vi "AVI Video Conditional Close.vi"(8 "error in (no error)":errorcluster, 11 "Logging queue element in":T1={"Imaging Protocol"=enum."Live Imaging", "Number of Trials"=0, "Frame Size"=512, "# Averaged frames"=0, "Dwell time (us)"=0.0, "Index of Z-plane"=0, "Timelapse?"=FALSE, "Logging process is active"=FALSE, "Speed logging enabled"=FALSE, "tdms file ref"=refnum, "path"=path "", "Trial Number"=0, "Expected # points acquired"=FALSE, "Manually stopped"=FALSE, "Last trial"=FALSE, "Ch0 data"=[], "Ch1 data"=[], "Ref Data"=[], "Ref Frame Time"=[], "Image Time"=[], "Continuous Time"=[], "Ref X Length"=0, "Ref Y Length"=0, "# Ref Averaged frames"=0, "Ref Dwell time (us)"=0.0, "Points acquired"={"Ch0 last trial"=0, "Ch1 last trial"=0, "All trials"=0}, "HW Timings File"=refnum} {"Ref Dwell time (us)" format="%#.6g"; "Frame Size" items=["100X100"=100, "128X128"=128, "200X200"=200, "256X256"=256, "512X512"=512, "1024x1024"=1024, "2048x2048"=2048]; "Dwell time (us)" format="%#.6g"}) -> (0 "error out":errorcluster)   [LabVIEW 2020]
uses:
  Typedefs/Logging queue element.ctl
  Typedefs/Imaging Protocols enum.ctl
  Typedefs/Frame Size.ctl
  Typedefs/Acquired points count.ctl
  Typedefs/Read Write Enum.ctl
  Globals/gl_Binary time series files globals.vi
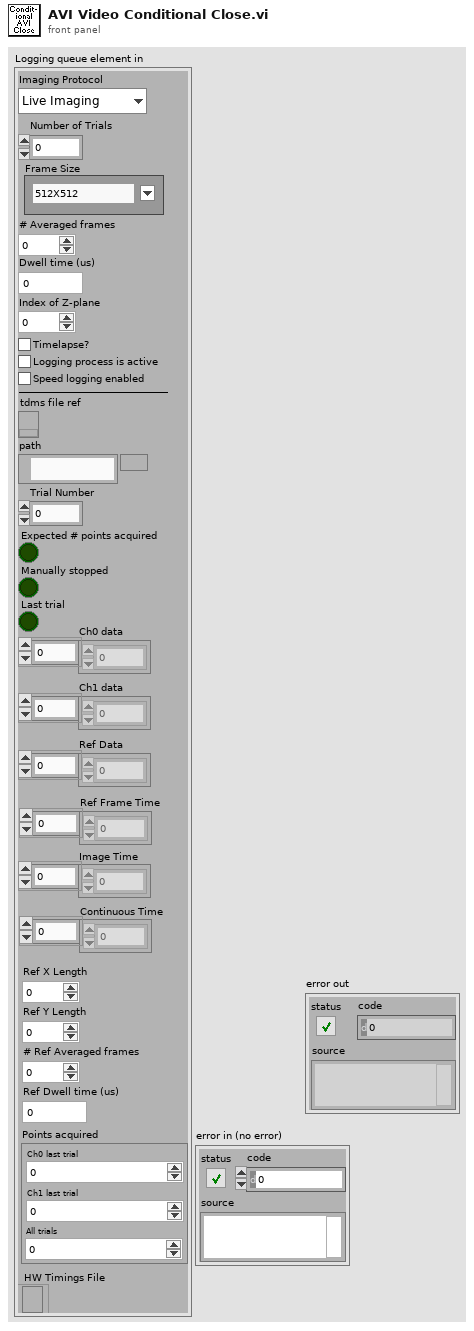
[diagram p1: front panel]
types:
  T1 = typedef "Logging queue element.ctl" = cluster{"Imaging Protocol":T2, "Number of Trials":u16, "Frame Size":T3, "# Averaged frames":u16, "Dwell time (us)":dbl, "Index of Z-plane":i32, "Timelapse?":bool, "Logging process is active":bool, "Speed logging enabled":bool, "tdms file ref":refnum<k34>, "path":path, "Trial Number":i32, "Expected # points acquired":bool, "Manually stopped":bool, "Last trial":bool, "Ch0 data":u32[], "Ch1 data":u32[], "Ref Data":u32[], "Ref Frame Time":u64[], "Image Time":u64[], "Continuous Time":u64[], "Ref X Length":u16, "Ref Y Length":u16, "# Ref Averaged frames":u16, "Ref Dwell time (us)":dbl, "Points acquired":T4, "HW Timings File":refnum<file>}
  T2 = typedef "Imaging Protocols enum.ctl" = enum16{"AOL Z-Stack", "Motor Z Stack", "Functional Acquisition", "Single Plane Acquisition", "Volume Acquisition", "Live Imaging", "Live Plane Imaging", "Live Volume Imaging"}
  T3 = typedef "Frame Size.ctl" = u16
  T4 = typedef "Acquired points count.ctl" = cluster{"Ch0 last trial":u64, "Ch1 last trial":u64, "All trials":u64}
  T5 = typedef "Read Write Enum.ctl" = enum16{"Read", "Write"}
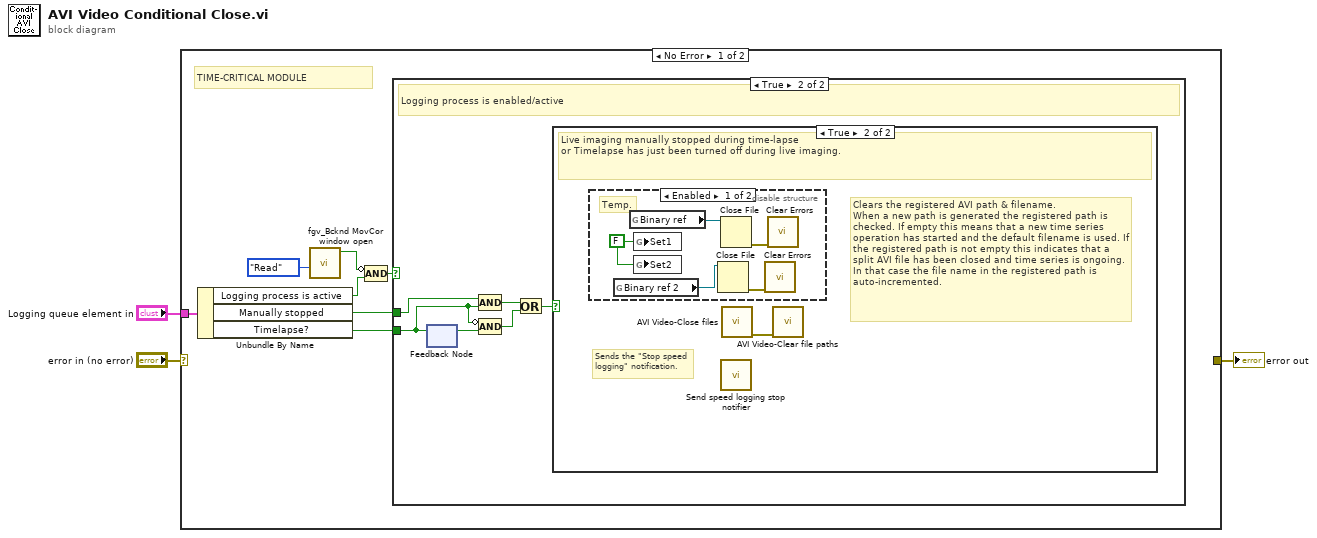
[diagram p0: block diagram]
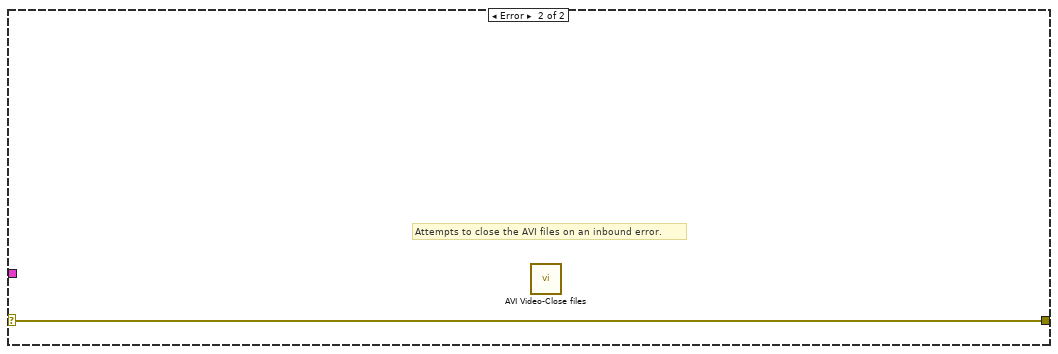
[diagram p5: hidden frame]
diagram:
  n1 = case shown="No Error" "error in (no error)" {
    selector: "error in (no error)" -> [_ w23]
    tunnel: "Logging queue element in" -> [w10 _]
    tunnel: [_ w23] -> w1
    frame No Error {
      # "TIME-CRITICAL MODULE"
      n2 = Unbundle By Name(w10) -> ("Logging process is active"=w7:bool, "Manually stopped"=w8:bool, "Timelapse?"=w9:bool)
      n3 = call "fgv_Bcknd MovCor window open.vi"("Function"=Read_Write_Enum."Read") -> ("Background MovCor window is open"=w4:bool)  [unwired: 9 in, 1 out]
      n4 = Compound Arithmetic op=AND(invert w4, w7) -> (w6:bool)
      n5 = case shown="True" w6 {
        tunnel: w9 -> [_ w13]
        tunnel: w8 -> [_ w12]
        frame False {
        }
        frame True {
          # "Logging process is enabled/active"
          n6 = feedback #1() -> (w15:bool)  [unwired: 1 in]
          n7 = feedback-in #1(w13) -> ()
          n8 = Compound Arithmetic op=AND(w12, w13) -> (w11:bool)
          n9 = Compound Arithmetic op=AND(invert w13, w15) -> (w14:bool)
          n10 = Or(x=w11, y=w14) -> (x .or. y?=w16:bool)
          n11 = case shown="True" w16 {
            frame False {
              # "Not stopped"
            }
            frame True {
              # "Sends the \"Stop speed logging\" notification."
              # "Clears the registered AVI path & filename.\nWhen a new path is generated the registered path is checked. If empty this means that a new time series operation has started and the default filename is used. If the registered path is not empty this indicates that a split AVI file has been closed and time series is ongoing. In that case the file name in the registered path is auto-incremented."
              # "Live imaging manually stopped during time-lapse\nor Timelapse has just been turned off during live imaging."
              n12 = disable-structure shown="Enabled" {
                frame Enabled {
                  w18 = FALSE ("Set1")
                  # "Temp."
                  n13 = global read "gl_Binary time series files globals.vi" "Binary ref 2"() -> (w19:refnum<file>)
                  n14 = global read "gl_Binary time series files globals.vi" "Binary ref"() -> (w22:refnum<file>)
                  n15 = global write "gl_Binary time series files globals.vi" "Set1"(w18) -> ()
                  n16 = global write "gl_Binary time series files globals.vi" "Set2"(w18) -> ()
                  n17 = Close File(refnum=w19) -> (error out=w20:errorcluster)  [unwired: 1 in, 1 out]
                  n18 = Close File(refnum=w22) -> (error out=w21:errorcluster)  [unwired: 1 in, 1 out]
                  n19 = call <vilib>:"Clear Errors.vi"("error in (no error)"=w20) -> ()  [unwired: 5 in, 2 out]
                  n20 = call <vilib>:"Clear Errors.vi"("error in (no error)"=w21) -> ()  [unwired: 5 in, 2 out]
                }
                frame Disabled {
                }
              }
              n21 = call "Send speed logging stop notifier.vi"() -> ()  [unwired: 11 in, 1 out]
              n22 = call "AVI Video-Close files.vi"() -> ("error out (pass through)"=w17:errorcluster)  [unwired: 11 in]
              n23 = call "AVI Video-Clear file paths.vi"("error in (no error)"=w17) -> ()  [unwired: 10 in, 1 out]
            }
          }
        }
      }
    }
    frame Error {
      # "Attempts to close the AVI files on an inbound error."
      n24 = call "AVI Video-Close files.vi"() -> ()  [unwired: 11 in, 1 out]
    }
  }
  "error out" <- w1
